vi "GetExecutionMode.vi"(8 "error in (no error)":errorcluster, 11 "absolute custom device xml file":path) -> (0 "error out":errorcluster, 2 "execution mode":T1, 3 "absolute custom device xml file":path)   [LabVIEW 2015, in "VeriStandTestCase.lvclass"]
uses:
  VeriStandTestCase.lvclass
  <vilib>/NI Veristand/Custom Device API/Custom Device Execution Mode.ctl
  <vilib>/xml/Load XML File.vi
  <vilib>/xml/Close Reference(Node).vi
  <vilib>/xml/NI_XML.lvlib
  <vilib>/NI Veristand/Custom Device API/Custom Device API.lvlib
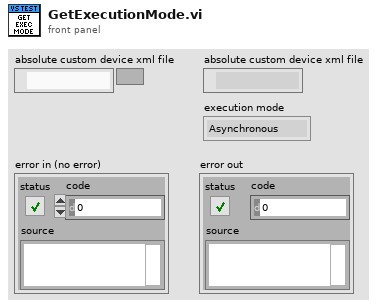
[diagram p1: front panel]
types:
  T1 = typedef "Custom Device API.lvlib/Custom Device Execution Mode.ctl" = enum16{"Asynchronous", "Inline HW Interface", "Inline Model Interface", "Inline Timing and Sync", "Asynchronous Timing and Sync"}
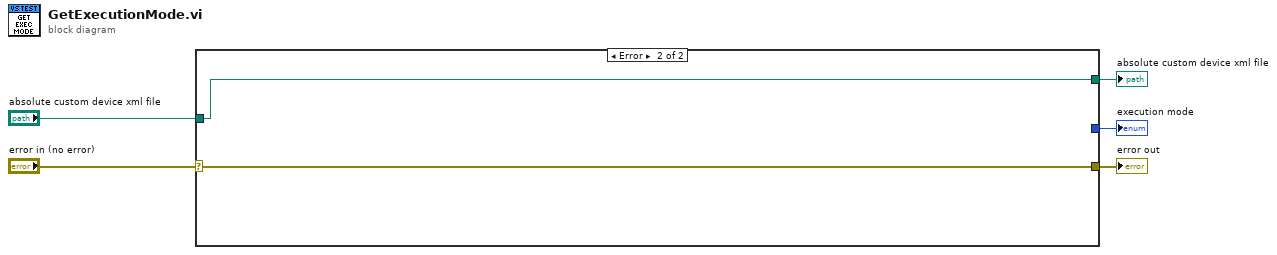
[diagram p0: block diagram]
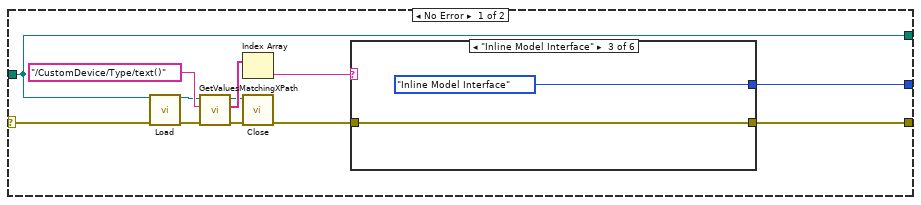
[diagram p2: hidden frame]
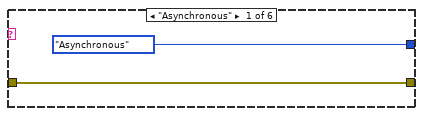
[diagram p3: hidden frame]
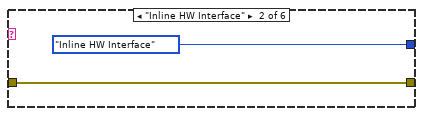
[diagram p4: hidden frame]
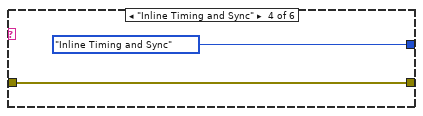
[diagram p5: hidden frame]
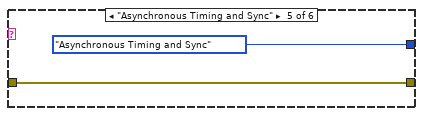
[diagram p6: hidden frame]
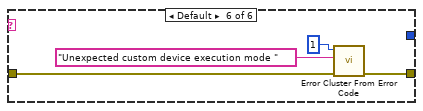
[diagram p7: hidden frame]
diagram:
  n1 = case shown="Error" "error in (no error)" {
    selector: "error in (no error)" -> [w17 w33]
    tunnel: "absolute custom device xml file" -> [w6 w32]
    tunnel: [w7 w33] -> w3
    tunnel: [w9 _] -> w2
    tunnel: [w6 w32] -> w1
    frame No Error {
      n2 = call-poly <vilib>:"Load.vi"("path to XML document"=w6, "error in (no error)"=w17) -> ("DOM document out"=w12:refnum<k20>, "error out"=w14:errorcluster)  [unwired: 11 in, 1 out]
      n3 = call "GetValuesMatchingXPath.vi"("error in (no error)"=w14, "XPath"="/CustomDevice/Type/text()", "XML refnum in"=w12) -> ("error out"=w15:errorcluster, "Values"=w13:string[], "XML refnum out"=w11:refnum<k20>)  [unwired: 6 in]
      n4 = Index Array(array=w13) -> (element=w10:string)  [unwired: 1 in]
      n5 = call-poly <vilib>:"Close.vi"("error in (no error)"=w15, "node"=w11) -> ("error out"=w8:errorcluster)  [unwired: 7 in]
      n6 = case shown="\"Inline Model Interface\"" w10 {
        tunnel: [Custom_Device_Execution_Mode."Asynchronous" ("Execution Mode") Custom_Device_Execution_Mode."Inline HW Interface" ("Execution Mode") Custom_Device_Execution_Mode."Inline Model Interface" ("Execution Mode") Custom_Device_Execution_Mode."Inline Timing and Sync" ("Execution Mode") Custom_Device_Execution_Mode."Asynchronous Timing and Sync" ("Execution Mode") _] -> w9
        tunnel: w8 -> [w18 w20 w22 w24 w26 w29]
        tunnel: [w18 w20 w22 w24 w26 w28] -> w7
        frame "Asynchronous" {
        }
        frame "Inline HW Interface" {
        }
        frame "Inline Model Interface" {
        }
        frame "Inline Timing and Sync" {
        }
        frame "Asynchronous Timing and Sync" {
        }
        frame Default {
          n7 = call <vilib>:"Error Cluster From Error Code.vi"("error in (no error)"=w29, "error message (\"\")"="Unexpected custom device execution mode " ("error message (\"\")"), "error code (0)"=1) -> ("error out"=w28:errorcluster)  [unwired: 6 in]
        }
      }
    }
    frame Error {
    }
  }
  "error out" <- w3
  "execution mode" <- w2
  "absolute custom device xml file" <- w1
